vi "DM3058 drive.vi"(6 "Function Choose":T2=enum."Measure", 8 "error in (no error)":errorcluster, 9 "parameter":T1={"Reset (True)"=TRUE, "ID Query (True)"=FALSE, "Auto Range (T:Enable)"=FALSE, "Function (0: DC Volts)"=0, "Range Select"=enum."20V", "Absolute Resolution (0: 5.5 Rate:Slow)"=0} {"Absolute Resolution (0: 5.5 Rate:Slow)" items=["5.5 Rate:Slow", "4.5 Rate:Middle", "4.5 Rate:Fast", "3.5 Rate", "6.5 Rate"]; "Function (0: DC Volts)" items=["DC Volts", "AC Volts", "DC Current", "AC Current", "2-Wire Resistance", "4-Wire Resistance", "Frequency", "Period", "Continuity", "Diode", "Capacitance", "Ratio"]}, 11 "VISA resource name":refnum<visa-resource-name>) -> (0 "error out":errorcluster, 2 "Measurement":dbl format="%#.6g", 3 "VISA resource name out":refnum<visa-resource-name>)   [LabVIEW 2020]
uses:
  subvi/DM3058 Function Choose.ctl
  <instrlib>/RIGOL DM3058/RIGOL DM3058.lvlib
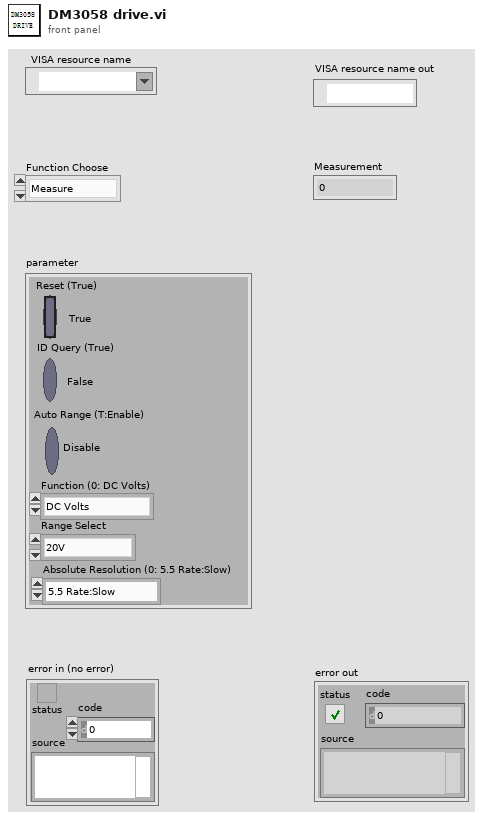
[diagram p1: front panel]
types:
  T1 = cluster{"Reset (True)":bool, "ID Query (True)":bool, "Auto Range (T:Enable)":bool, "Function (0: DC Volts)":u16, "Range Select":enum16{"200mV", "2V", "20V", "200V", "1000V"}, "Absolute Resolution (0: 5.5 Rate:Slow)":u16}
  T2 = typedef "DM3058 Function Choose.ctl" = enum16{"Close", "Measure", "Config", "Init"}
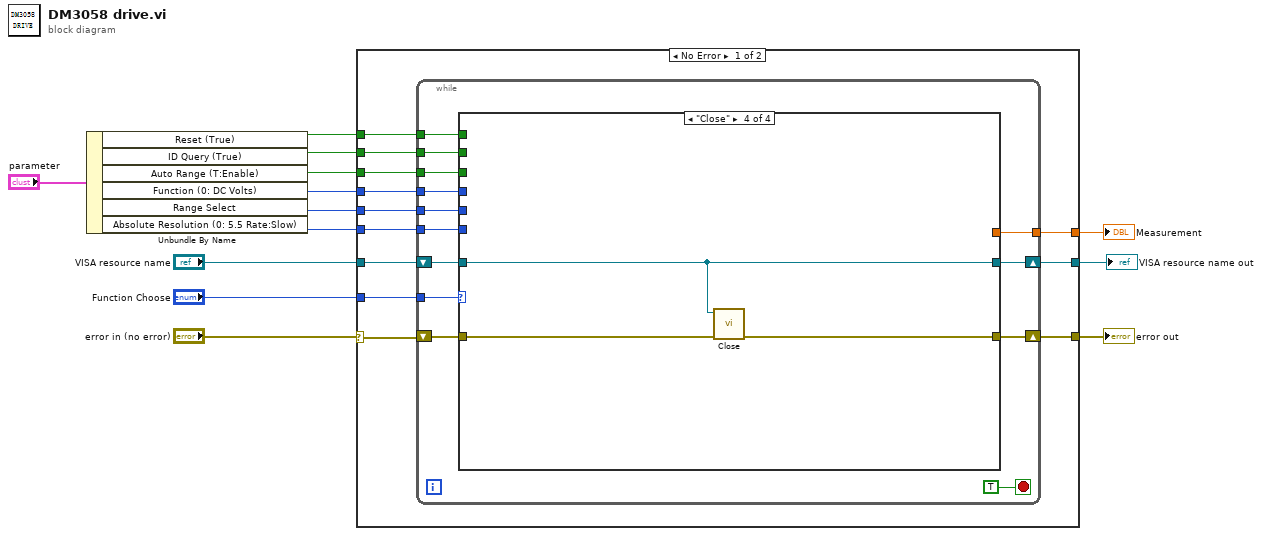
[diagram p0: block diagram]
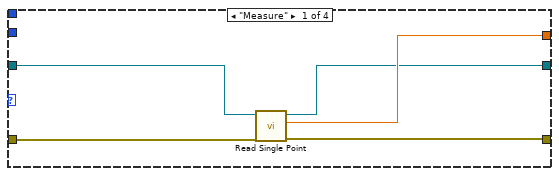
[diagram p2: hidden frame]
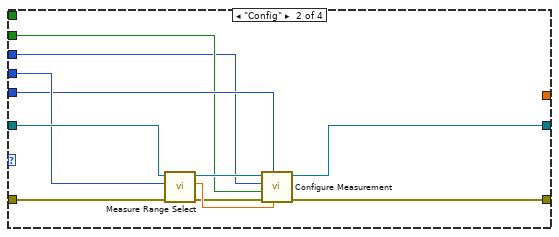
[diagram p3: hidden frame]
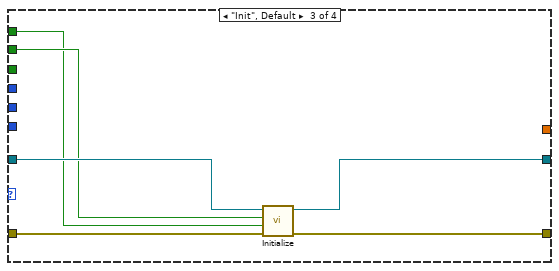
[diagram p4: hidden frame]
diagram:
  n1 = Unbundle By Name("parameter") -> ("Reset (True)"=w5:bool, "ID Query (True)"=w6:bool, "Auto Range (T:Enable)"=w2:bool, "Function (0: DC Volts)"=w1:u16, "Range Select"=w4:enum16{"200mV", "2V", "20V", "200V", "1000V"}, "Absolute Resolution (0: 5.5 Rate:Slow)"=w3:u16)
  n2 = case shown="No Error" "error in (no error)" {
    selector: "error in (no error)" -> [w20 w64]
    tunnel: "Function Choose" -> [w25 _]
    tunnel: "VISA resource name" -> [w24 _]
    tunnel: [w23 w64] -> w11
    tunnel: [w22 _] -> w10
    tunnel: [w21 _] -> w9
    tunnel: w6 -> [w19 _]
    tunnel: w5 -> [w18 _]
    tunnel: w4 -> [w17 _]
    tunnel: w3 -> [w16 _]
    tunnel: w2 -> [w15 _]
    tunnel: w1 -> [w14 _]
    frame No Error {
      n3 = while {
        tunnel: w25 -> [w38]
        shift-right: [w34] -> w22
        shift-left: w24 -> [w37]
        shift-right: [w36] -> w23
        shift-left: w20 -> [w35]
        tunnel: [w32] -> w21
        tunnel: w19 -> [w31]
        tunnel: w18 -> [w30]
        tunnel: w17 -> [w29]
        tunnel: w16 -> [w28]
        tunnel: w15 -> [w27]
        tunnel: w14 -> [w26]
        stop <- TRUE stop-if-true
        n4 = case shown="\"Close\"" w38 {
          tunnel: w37 -> [w42 w49 w60 w61]
          tunnel: [w40 w54 w58 w62] -> w36
          tunnel: w35 -> [w41 w51 w59 w63]
          tunnel: [w43 _ _ _] -> w32
          tunnel: [w39 w53 w57 w61] -> w34
          tunnel: w31 -> [_ _ w56 _]
          tunnel: w30 -> [_ _ w55 _]
          tunnel: w29 -> [_ w47 _ _]
          tunnel: w28 -> [_ w46 _ _]
          tunnel: w27 -> [_ w45 _ _]
          tunnel: w26 -> [_ w44 _ _]
          frame "Measure" {
            n5 = call <instrlib>:"Read Single Point.vi"("error in (no error)"=w41, "VISA resource name"=w42) -> ("error out"=w40:errorcluster, "Measurement"=w43:dbl, "VISA resource name out"=w39:refnum<visa-resource-name>)  [unwired: 7 in]
          }
          frame "Config" {
            n6 = call "Measure Range Select.vi"("error in (no error)"=w51, "Range Select"=w47, "VISA resource name"=w49) -> ("error out"=w50:errorcluster, "Numeric"=w52:dbl, "VISA resource out"=w48:refnum<visa-resource-name>)  [unwired: 6 in]
            n7 = call <instrlib>:"Configure Measurement.vi"("Manual Range (1.00)"=w52, "Absolute Resolution (0: 5.5 Rate:Slow)"=w46, "error in (no error)"=w50, "Auto Range (T:Enable)"=w45, "Function (0: DC Volts)"=w44, "VISA resource name"=w48) -> ("error out"=w54:errorcluster, "VISA resource name out"=w53:refnum<visa-resource-name>)  [unwired: 4 in]
          }
          frame "Init", Default {
            n8 = call <instrlib>:"Initialize.vi"("error in (no error)"=w59, "Reset (True)"=w55, "ID Query (True)"=w56, "VISA resource name"=w60) -> ("error out"=w58:errorcluster, "VISA resource name out"=w57:refnum<visa-resource-name>)  [unwired: 6 in]
          }
          frame "Close" {
            n9 = call <instrlib>:"Close.vi"("error in (no error)"=w63, "VISA resource name"=w61) -> ("error out"=w62:errorcluster)  [unwired: 9 in]
          }
        }
      }
    }
    frame Error {
    }
  }
  "error out" <- w11
  "Measurement" <- w9
  "VISA resource name out" <- w10
